vi "Pickup Up State.vi"(11 "Trigger":bool) -> ()   [LabVIEW 2013]
uses:
  Control 2.ctl
  <vilib>/Rock Robotics/WPI/Solenoid/Deprecated/WPI_SolenoidSetBool.vi
panel:
  out "Wait":bool
  out "Boolean":bool
  out "Elapsed Time (s) 2":dbl caption="Elapsed Time (s)"
  out "Arm Up":bool
  out "Clamp Close":bool
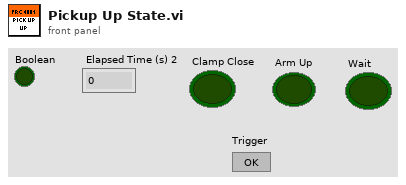
[diagram p1: front panel]
types:
  T1 = typedef "Control 2.ctl" = enum16{"Clamp Open", "Arm Up", "Wait"}
  T2 = typedef "WPI_SolenoidDevRef.ctl" = cluster{"DevStatus":errorcluster, "Solenoid Module":T3, "Forward Solenoid Channel":T4, "Reverse Solenoid Channel":T4}
  T3 = typedef "FPGA_TypedefSolenoidModule.ctl" = enum16{"Solenoid Module 1", "Solenoid Module 2"}
  T4 = typedef "WPI_SolenoidChannel.ctl" = enum8{"Solenoid 1", "Solenoid 2", "Solenoid 3", "Solenoid 4", "Solenoid 5", "Solenoid 6", "Solenoid 7", "Solenoid 8", "Invalid"}
  T5 = typedef "WPI_MotorControlDeviceRef.ctl" = cluster{"DeviceStatus":errorcluster, "Type":enum16{"PWM", "CAN"}, "PWM":cluster{"Digital Module":T6, "PWM Channel":T7, "DeadBand":T8}, "CAN":cluster{"Device Number":u8, "Control Mode":T9, "Semaphore":T10, "Max Vout":dbl}, "Invert":bool, "TransformRef":T11, "InvTransformRef":T11}
  T6 = typedef "FPGA_TypedefDigitalModule.ctl" = enum16{"Digital Module 1", "Digital Module 2"}
  T7 = typedef "FPGA_DIOPWMChannel.ctl" = enum8{"PWM 1", "PWM 2", "PWM 3", "PWM 4", "PWM 5", "PWM 6", "PWM 7", "PWM 8", "PWM 9", "PWM 10", "Invalid"}
  T8 = typedef "WPI_PWMDeadband.ctl" = cluster{"Name":string, "maxPositivePwm":i32, "minPositivePwm":i32, "centerPwm":i32, "maxNegativePwm":i32, "minNegativePwm":i32, "angularRange":u16}
  T9 = typedef "WPI_CANJaguar_ControlMode.ctl" = enum8{"Percent VBus", "Current", "Speed", "Position", "Voltage"}
  T10 = typedef "Semaphore RefNum" = refnum<k1>
  T11 = typedef "WPI_PWMTransform_ConPane.ctl" = refnum<vi>
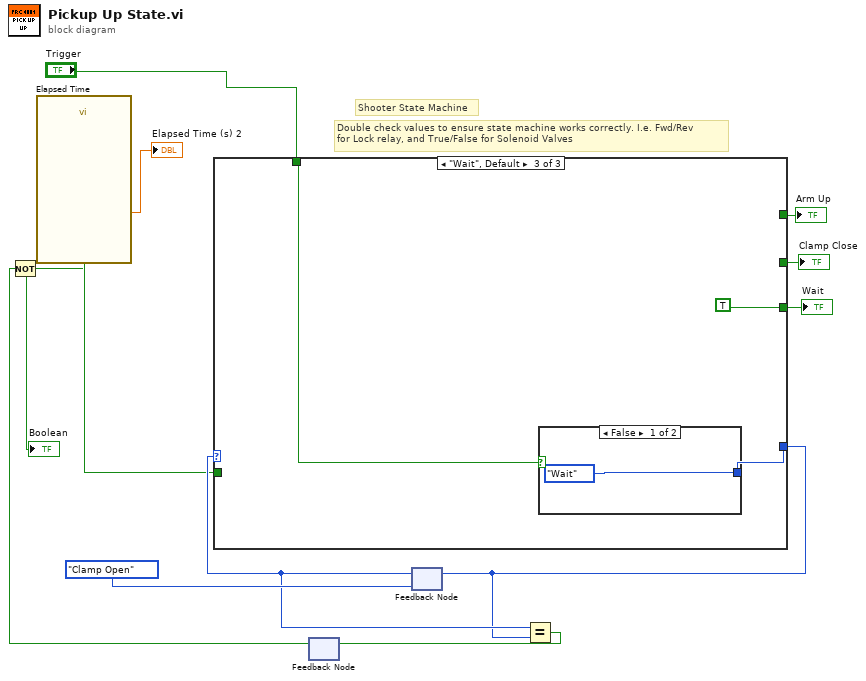
[diagram p0: block diagram]
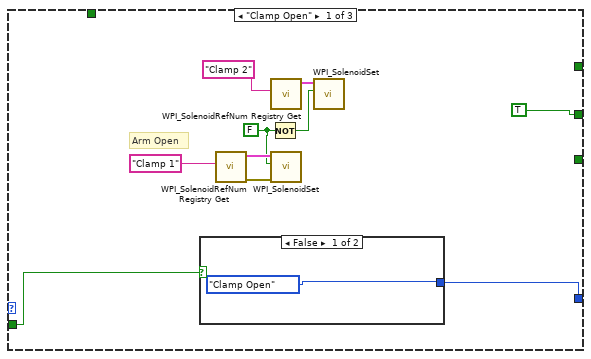
[diagram p2: hidden frame]
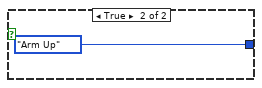
[diagram p3: hidden frame]
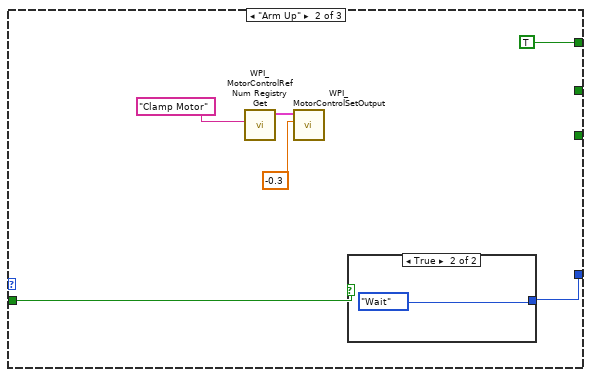
[diagram p4: hidden frame]
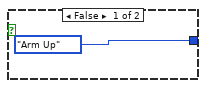
[diagram p5: hidden frame]
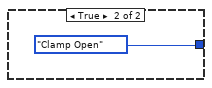
[diagram p6: hidden frame]
diagram:
  # "Double check values to ensure state machine works correctly. I.e. Fwd/Rev\nfor Lock relay, and True/False for Solenoid Valves"
  # "Shooter State Machine"
  n1 = feedback #1() -> (w5:bool)  [unwired: 1 in]
  n2 = Not(x=w5) -> (.not. x?=w3:bool)
  "Boolean" <- w3
  n3 = call "Elapsed Time"("Reset"=w3) -> ("Elapsed Time (s)"=→"Elapsed Time (s) 2":dbl, "Time has Elapsed"=w4:bool)  [unwired: 11 in, 6 out]
  n4 = feedback #2(Control_2."Clamp Open") -> (w9:T1)
  n5 = case shown="\"Wait\", Default" w9 {
    tunnel: [w22 w30 w35] -> w8
    tunnel: [TRUE ("State 0") _ _] -> w11
    tunnel: [_ TRUE _] -> w10
    tunnel: w4 -> [w13 w28 _]
    tunnel: "Trigger" -> [_ _ w33]
    tunnel: [_ _ TRUE] -> w1
    frame "Clamp Open" {
      w14 = FALSE ("x")
      # "Arm Open"
      n6 = case shown="False" w13 {
        tunnel: [Control_2."Clamp Open" Control_2."Arm Up"] -> w22
        frame False {
        }
        frame True {
        }
      }
      n7 = call <vilib>:"WPI_SolenoidRefNum Registry Get.vi"("refnum name"="Clamp 1") -> ("error out"=w18:errorcluster, "SolenoidDevRef"=w19:T2)  [unwired: 9 in]
      n8 = Not(x=w14) -> (.not. x?=w15:bool)
      n9 = call <vilib>:"WPI_SolenoidRefNum Registry Get.vi"("refnum name"="Clamp 2") -> ("SolenoidDevRef"=w17:T2)  [unwired: 9 in, 1 out]
      n10 = call-poly <vilib>:"WPI_SolenoidSet.vi"("error in (no error)"=w18, "Value"=w14, "SolenoidDevRef"=w19) -> ()  [unwired: 7 in, 2 out]
      n11 = call-poly <vilib>:"WPI_SolenoidSet.vi"("Value"=w15, "SolenoidDevRef"=w17) -> ()  [unwired: 8 in, 2 out]
    }
    frame "Arm Up" {
      n12 = call <vilib>:"WPI_MotorControlRefNum Registry Get.vi"("refnum name"="Clamp Motor") -> ("MotorControlDevRef"=w26:T5)  [unwired: 9 in, 1 out]
      n13 = call <vilib>:"WPI_MotorControlSetOutput.vi"("Output"=-0.3, "MotorControlDevRef"=w26) -> ()  [unwired: 7 in, 3 out]
      n14 = case shown="True" w28 {
        tunnel: [Control_2."Arm Up" Control_2."Wait"] -> w30
        frame False {
        }
        frame True {
        }
      }
    }
    frame "Wait", Default {
      n15 = case shown="False" w33 {
        tunnel: [Control_2."Wait" Control_2."Clamp Open"] -> w35
        frame False {
        }
        frame True {
        }
      }
    }
  }
  "Clamp Close" <- w11
  "Arm Up" <- w10
  "Wait" <- w1
  n16 = feedback-in #2(w8) -> ()
  n17 = Equal?(x=w9, y=w8) -> (x = y?=w6:bool)
  n18 = feedback-in #1(w6) -> ()
